vi "LVClass_HasoSlopes ctor from Image.vi"(0 "HasoSlopes (const)":refnum<class "HasoSlopes.lvclass">, 5 "Image":refnum<class "Image.lvclass">, 7 "Haso configuration file":path, 9 "start subpupil":T1, 11 "error in (no error)":errorcluster, 12 "check_calibration_checksum":bool) -> (4 "HasoSlopes (new)":refnum<class "HasoSlopes.lvclass">, 6 "Image (dup)":refnum<class "Image.lvclass">, 15 "error out":errorcluster)   [LabVIEW 2020, in "HasoSlopes.lvclass"]
doc: "HasoSlopes constructor from Image.\n\n<B>HasoSlopesIn</B> : Constant Pointer to HasoSlopes object.\n<B>HasoSlopesOut</B> : Constant Pointer to HasoSlopes object.\n<B>Image</B> : Image object.\n<B>config_file_path</B> : Absolute path to Haso configuration file.\n<B>start_subpupil</B> : Coordinates of the first calculated sub-pupil (index coordinates relative to\n the top-left corner of the pupil).\n<B>check_calibration_checksum</B> : activation of the calibration checksum verification."
uses:
  HasoSlopes.lvclass
  Image.lvclass
  Point2D.ctl
  Handle creation.ctl
  HasoSlopes.lvclass/HasoSlopes.ctl
  LVClass_Image Read Image.vi
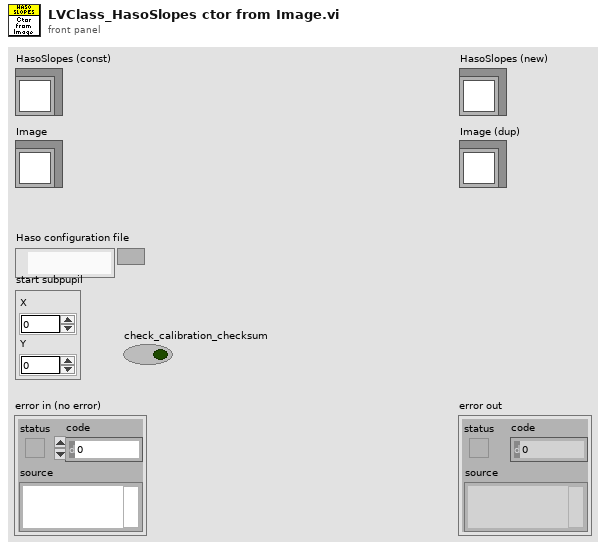
[diagram p1: front panel]
types:
  T1 = typedef "Point2D.ctl" = cluster{"X":u32, "Y":u32}
  T2 = typedef "Handle creation.ctl" = enum16{"By ctor", "By write function"}
  T3 = typedef "Struct_Image.ctl" = cluster{"Image_Handler":T4, "Number of bits":T5, "ImageSize":T1}
  T4 = typedef "ClassID.ctl" = i64
  T5 = typedef "Data alignment enum.ctl" = enum16{"8", "16", "32"}
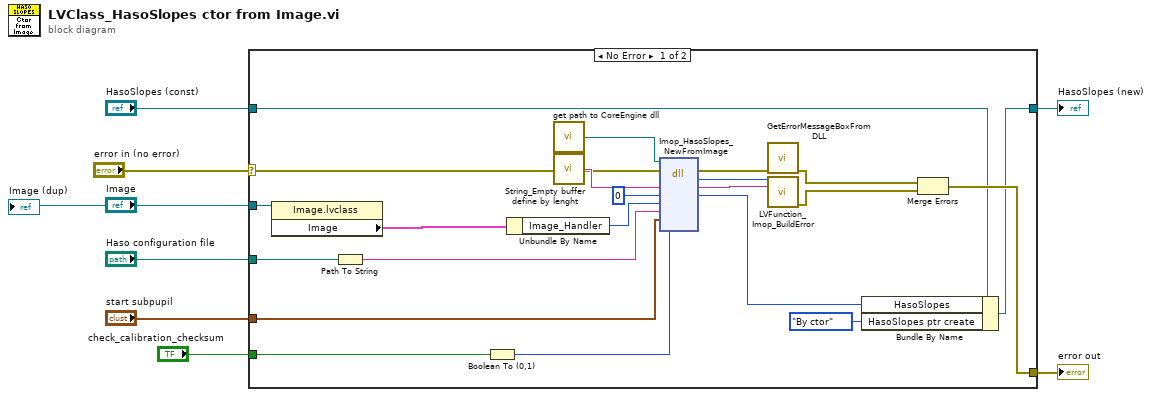
[diagram p0: block diagram]
diagram:
  n1 = case shown="No Error" "error in (no error)" {
    selector: "error in (no error)" -> [w23 w32]
    tunnel: [w22 w32] -> w7
    tunnel: [w20 w31] -> w5
    tunnel: "HasoSlopes (const)" -> [w21 w31]
    tunnel: "Image" -> [w17 _]
    tunnel: "Haso configuration file" -> [w14 _]
    tunnel: "start subpupil" -> [w11 _]
    tunnel: "check_calibration_checksum" -> [w9 _]
    frame No Error {
      n2 = property class="Image.lvclass"(reference=w17) -> ("Image"=w16:T3)  [unwired: 1 in, 2 out]
      n3 = Path To String(path=w14) -> (string=w13:string)
      n4 = Boolean To (0,1)(Boolean=w9) -> (0, 1=w10:i16)
      n5 = Unbundle By Name(w16) -> ("Image_Handler"=w15:T4)
      n6 = call "get path to CoreEngine dll.vi"() -> ("path to wavekit library"=w26:path)  [unwired: 14 in, 1 out]
      n7 = call "String_Empty buffer define by lenght.vi"() -> ("Empty buffer"=w27:string)  [unwired: 1 in]
      n8 = dll-call lib="D:/FLE/0.Code/CoreEngine4_Suite/LV2011_interface/DLLs/c_interface_vc100.dll" fn="Imop_HasoSlopes_NewFromImage"(path in=w26, error in=w23, "Message"=w27, "HasoSlopes"=0, "Image"=w15, "HASO configuration path"=w13, "start subpupil"=w11, "check_calibration_checksum"=w10) -> (error out=w30:errorcluster, "return type"=w28:i32, "Message"=w29:string, "HasoSlopes"=w12:i64)  [unwired: 5 in, 1 out]
      n9 = call "GetErrorMessageBoxFromDLL.vi"("error IN"=w30) -> ("error OUT"=w25:errorcluster)  [unwired: 10 in]
      n10 = call "LVFunction_Imop_BuildError.vi"("code"=w28, "String to Prepend to source (\"\")"=w29) -> ("error out"=w24:errorcluster)  [unwired: 13 in]
      n11 = Bundle By Name(cluster=w21, "HasoSlopes"=w12, "HasoSlopes ptr create"=Handle_creation."By ctor") -> (w20:refnum<class "HasoSlopes.lvclass">)
      n12 = Merge Errors(w25, w24) -> (w22:errorcluster)
    }
    frame Error {
    }
  }
  "error out" <- w7
  "HasoSlopes (new)" <- w5
  "Image (dup)" <- "Image"
